vi "设置电压模块窗口.vi"() -> (0 "打开/关闭":bool, 1 "确定输出":bool)   [LabVIEW 2016, in "ADCP.lvlib"]
uses:
  ADCP.lvlib
  <vilib>/Utility/config.llb/NI_LVConfig.lvlib
panel:
  in  "量程写入":bool
  in  "量程上限":i16=9999
  in  "量程下限":i16
  in  "串口":refnum<visa-resource-name>="COM6"
  in  "串口开关":bool
  in  "取消":bool
  in  "确定":bool
  # "设置电压模块参数"
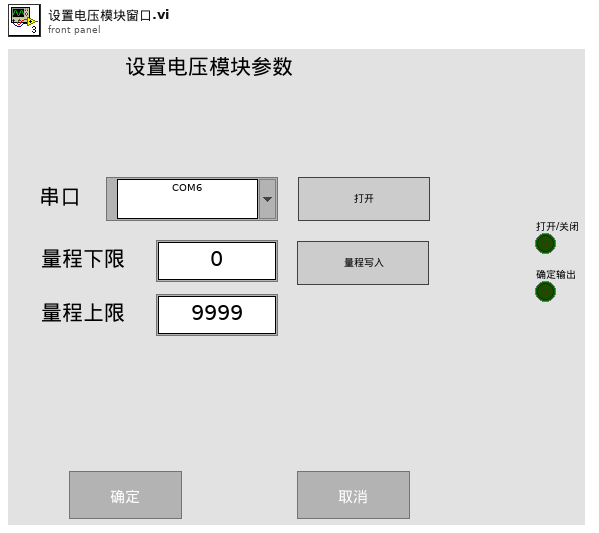
[diagram p1: front panel]
types:
  T1 = typedef "NI_LVConfig.lvlib/Config Data RefNum.ctl" = refnum<k1>
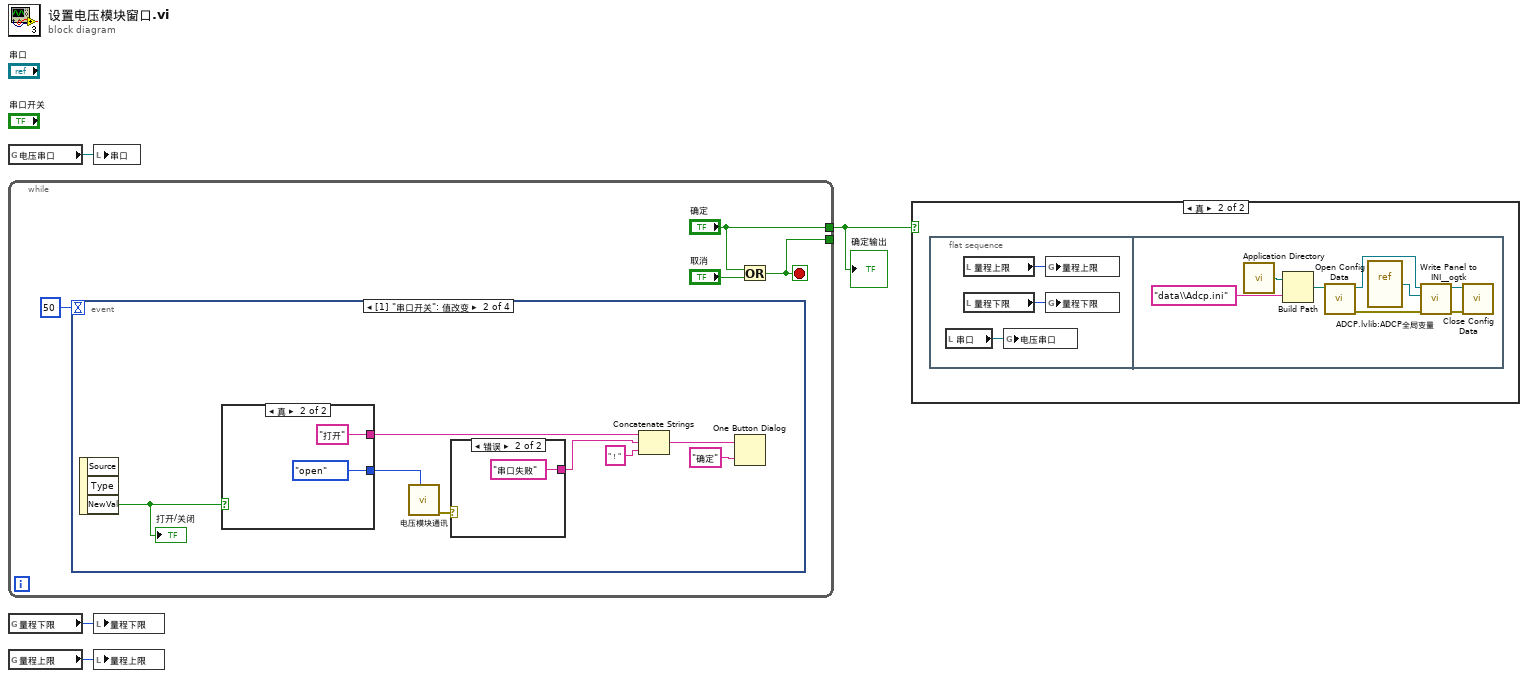
[diagram p0: block diagram]
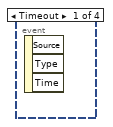
[diagram p3: hidden frame]
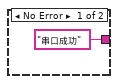
[diagram p4: hidden frame]
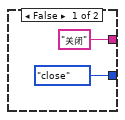
[diagram p5: hidden frame]
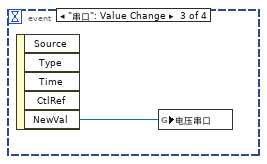
[diagram p6: hidden frame]
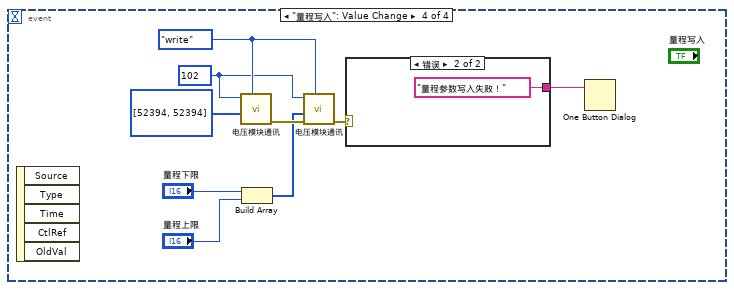
[diagram p7: hidden frame]
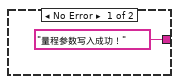
[diagram p8: hidden frame]
diagram:
  n1 = global read "ADCP全局变量.vi" "电压串口"() -> (w4:refnum<visa-resource-name>)
  n2 = while {
    tunnel: [w6] -> _
    tunnel: ["确定"] -> w3
    stop <- w6 stop-if-true
    n3 = event shown="[1] \"串口开关\": 值改变" {
      selector: _ -> [_ _ _ _]
      dyn-events: _ -> [_ _ _ _]
      timeout: 50 -> [_ _ _ _]
      event Timeout {
        n4 = event-data() -> ()  [unwired: 1 in, 3 out]
      }
      event "串口开关": Value Change {
        n5 = event-data() -> ("NewVal"=w16:bool)  [unwired: 1 in, 2 out]
        "打开/关闭" <- w16
        n6 = case shown="真" w16 {
          tunnel: [enum16{"open", "read", "write", "close"}."close" ("STEP") enum16{"open", "read", "write", "close"}."open" ("STEP")] -> w15
          tunnel: ["关闭" "打开"] -> w13
          frame False {
          }
          frame True {
          }
        }
        n7 = call "电压模块通讯.vi"("STEP"=w15) -> ("error out"=w14:errorcluster)  [unwired: 8 in, 2 out]
        n8 = case shown="错误" w14 {
          tunnel: ["串口成功" "串口失败"] -> w9
          frame No Error {
          }
          frame Error {
          }
        }
        n9 = Concatenate Strings(w13, w9, "！" ("字符串")) -> (w11:string)
        n10 = One Button Dialog(message=w11, button name ("OK")="确定" ("按钮名称（“确定”）")) -> ()  [unwired: 1 out]
      }
      event "串口": Value Change {
        n11 = event-data() -> ("NewVal"=w23:refnum<visa-resource-name>)  [unwired: 1 in, 4 out]
        n12 = global write "ADCP全局变量.vi" "电压串口"(w23) -> ()
      }
      event "量程写入": Value Change {
        w30 = u16 102 ("address")
        w31 = enum16{"open", "read", "write", "close"}."write" ("STEP")
        n13 = event-data() -> ()  [unwired: 1 in, 5 out]
        n14 = call "电压模块通讯.vi"("STEP"=w31, "values"=u16[] [52394, 52394], "starting address"=w30) -> ("error out"=w32:errorcluster)  [unwired: 6 in, 2 out]
        n15 = Build Array("量程下限", "量程上限") -> (w28:i16[])
        n16 = call "电压模块通讯.vi"("STEP"=w31, "Error in"=w32, "values"=w28, "starting address"=w30) -> ("error out"=w25:errorcluster)  [unwired: 5 in, 2 out]
        n17 = case shown="错误" w25 {
          tunnel: ["量程参数写入成功！" ("消息") "量程参数写入失败！" ("消息")] -> w24
          frame No Error {
          }
          frame Error {
          }
        }
        n18 = One Button Dialog(message=w24) -> ()  [unwired: 1 in, 1 out]
      }
    }
    n19 = Or(x="确定", y="取消") -> (x .or. y?=w6:bool)
  }
  "确定输出" <- w3
  n20 = global read "ADCP全局变量.vi" "量程下限"() -> (w1:i16)
  n21 = global read "ADCP全局变量.vi" "量程上限"() -> (w2:i16)
  n22 = local write "串口"(w4) -> ()
  n23 = local write "量程下限"(w1) -> ()
  n24 = local write "量程上限"(w2) -> ()
  n25 = case shown="真" w3 {
    frame False {
    }
    frame True {
      n26 = flat-sequence {
        frame #0 {
          n27 = local read "串口"() -> (w37:refnum<visa-resource-name>)
          n28 = local read "量程上限"() -> (w35:i16)
          n29 = local read "量程下限"() -> (w36:i16)
          n30 = global write "ADCP全局变量.vi" "电压串口"(w37) -> ()
          n31 = global write "ADCP全局变量.vi" "量程上限"(w35) -> ()
          n32 = global write "ADCP全局变量.vi" "量程下限"(w36) -> ()
        }
        frame #1 {
          n33 = call <vilib>:"Application Directory.vi"() -> ("Application Directory"=w41:path)
          n34 = Build Path(base path=w41, name or relative path="data\\Adcp.ini" ("名称或相对路径")) -> (appended path=w43:path)
          n35 = call <vilib>:"Open Config Data.vi"("configuration file path"=w43) -> ("error out"=w39:errorcluster, "refnum"=w44:T1)  [unwired: 8 in, 1 out]
          n36 = vi-ref "ADCP.lvlib:ADCP全局变量.vi"() -> (w38:refnum<vi>)
          n37 = call <userlib>:"Write Panel to INI__ogtk.vi"("error in (no error)"=w39, "VI ref"=w38, "refnum"=w44) -> ("error out"=w40:errorcluster, "refnum out"=w45:T1)  [unwired: 7 in]
          n38 = call <vilib>:"Close Config Data.vi"("error in (no error)"=w40, "refnum"=w45) -> ()  [unwired: 8 in, 2 out]
        }
      }
    }
  }
